vi "Ustaw wspolne.vi"(7 "WaveformGraph in":refnum<vi>, 8 "error in (no error)":errorcluster, 10 "Bounds":T2, 11 "Array":refnum<vi>[](array[refnum])) -> (0 "error out":errorcluster, 2 "Pos Array":T1[](array[typedef]))   [LabVIEW 2014]
doc: "Ustawia wspólne elementy okien Rejestracja szybka i rejestracja wolna."
uses:
  <vilib>/Utility/miscctls.llb/LVBoundsTypeDef.ctl
  <vilib>/Utility/miscctls.llb/LVPositionTypeDef.ctl
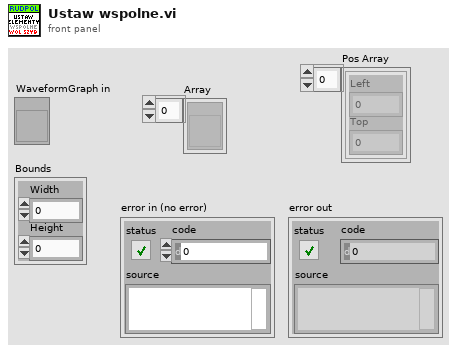
[diagram p1: front panel]
types:
  T1 = typedef "LVPositionTypeDef.ctl" = cluster{"Left":i32, "Top":i32}
  T2 = typedef "LVBoundsTypeDef.ctl" = cluster{"Width":u32, "Height":u32}
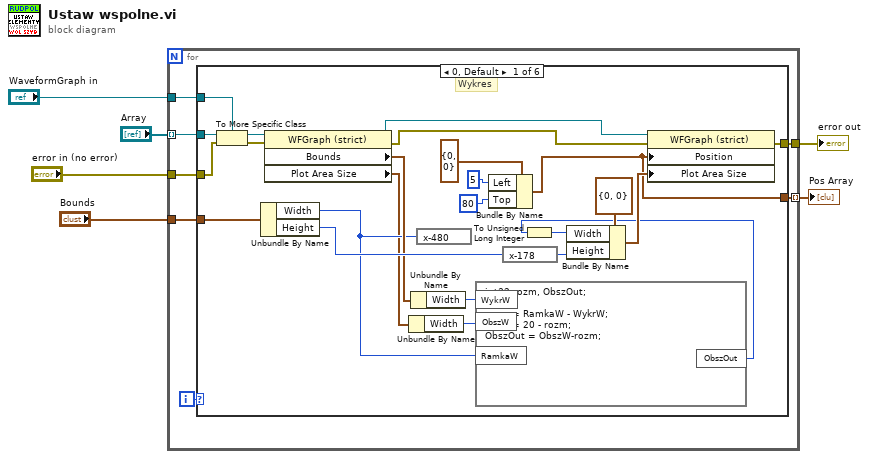
[diagram p0: block diagram]
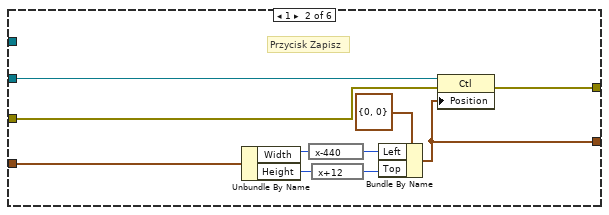
[diagram p2: hidden frame]
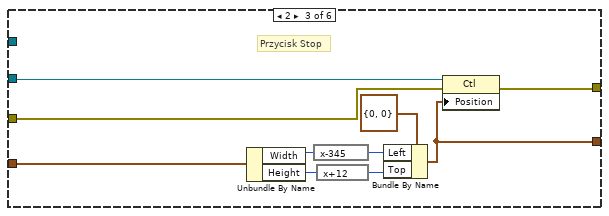
[diagram p3: hidden frame]
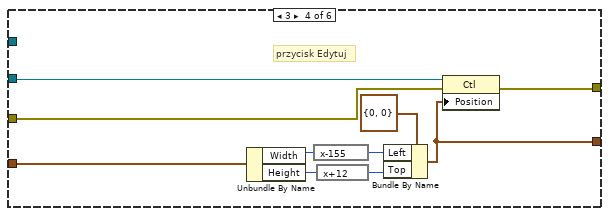
[diagram p4: hidden frame]
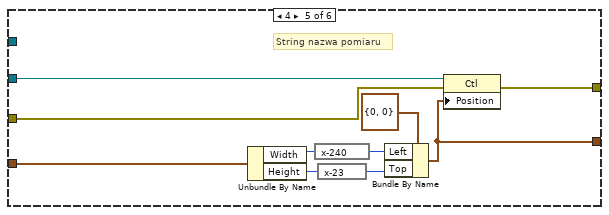
[diagram p5: hidden frame]
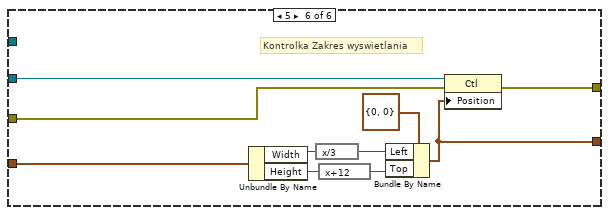
[diagram p6: hidden frame]
diagram:
  n1 = for {
    tunnel: "Array" -> [w12] mode=indexing
    tunnel: "Bounds" -> [w11]
    tunnel: "WaveformGraph in" -> [w10]
    tunnel: [w9] -> w3 mode=indexing
    tunnel: "error in (no error)" -> [w8]
    tunnel: [w7] -> w1
    i -> [w13]
    n2 = case shown="0, Default" w13 {
      tunnel: w12 -> [w34 w47 w52 w62 w72 w82]
      tunnel: w11 -> [w32 w45 w51 w61 w71 w81]
      tunnel: w10 -> [w33 _ _ _ _ _]
      tunnel: [w27 w40 w50 w60 w70 w80] -> w9
      tunnel: w8 -> [w25 w38 w48 w58 w68 w79]
      tunnel: [w26 w39 w49 w59 w69 w78] -> w7
      frame 0, Default {
        # "Wykres"
        n3 = To More Specific Class(target class=w33, reference=w34, error in=w25) -> (specific class reference=w23:refnum<vi>, error out=w24:errorcluster)
        n4 = Unbundle By Name(w32) -> ("Width"=w16:u32, "Height"=w30:u32)
        n5 = property class="WFGraph (strict)"(reference=w23, error in=w24) -> (reference out=w21:refnum<vi>, error out=w22:errorcluster, "Bounds"=w20:T2, "Plot Area Size"=w14:T2)
        n6 = Unbundle By Name(w14) -> ("Width"=w15:u32)
        n7 = Unbundle By Name(w20) -> ("Width"=w19:u32)
        n8 = expression code="x-480"(w16) -> ()  [unwired: 1 out]
        n9 = formula code="int32 rozm, ObszOut;\n\nrozm = RamkaW - WykrW;\nrozm = 20 - rozm;\nObszOut = ObszW-rozm;"("RamkaW"=w16, "WykrW"=w19, "ObszW"=w15) -> ("ObszOut"=w18:i32)
        n10 = Bundle By Name(cluster=T1 {"Left"=0, "Top"=0} ("Position"), "Left"=5 ("y"), "Top"=80 ("y")) -> (w27:T1)
        n11 = expression code="x-178"(w30) -> (w29:u32)
        n12 = To Unsigned Long Integer(number=w18) -> (unsigned 32bit integer=w17:u32)
        n13 = Bundle By Name(cluster=T2 {"Width"=0, "Height"=0} ("Plot Area:Size"), "Width"=w17, "Height"=w29) -> (w28:T2)
        n14 = property class="WFGraph (strict)"(reference=w21, error in=w22, "Position"=w27, "Plot Area Size"=w28) -> (error out=w26:errorcluster)  [unwired: 1 out]
      }
      frame 1 {
        # "Przycisk Zapisz"
        n15 = Unbundle By Name(w45) -> ("Width"=w44:u32, "Height"=w41:u32)
        n16 = expression code="x-440"(w44) -> (w43:u32)
        n17 = expression code="x+12"(w41) -> (w42:u32)
        n18 = Bundle By Name(cluster=T1 {"Left"=0, "Top"=0} ("Position"), "Left"=w43, "Top"=w42) -> (w40:T1)
        n19 = property class="Ctl"(reference=w47, error in=w38, "Position"=w40) -> (error out=w39:errorcluster)  [unwired: 1 out]
      }
      frame 2 {
        # "Przycisk Stop"
        n20 = Unbundle By Name(w51) -> ("Width"=w56:u32, "Height"=w53:u32)
        n21 = expression code="x-345"(w56) -> (w55:u32)
        n22 = expression code="x+12"(w53) -> (w54:u32)
        n23 = Bundle By Name(cluster=T1 {"Left"=0, "Top"=0} ("Position"), "Left"=w55, "Top"=w54) -> (w50:T1)
        n24 = property class="Ctl"(reference=w52, error in=w48, "Position"=w50) -> (error out=w49:errorcluster)  [unwired: 1 out]
      }
      frame 3 {
        # "przycisk Edytuj"
        n25 = Unbundle By Name(w61) -> ("Width"=w66:u32, "Height"=w63:u32)
        n26 = expression code="x-155"(w66) -> (w65:u32)
        n27 = expression code="x+12"(w63) -> (w64:u32)
        n28 = Bundle By Name(cluster=T1 {"Left"=0, "Top"=0} ("Position"), "Left"=w65, "Top"=w64) -> (w60:T1)
        n29 = property class="Ctl"(reference=w62, error in=w58, "Position"=w60) -> (error out=w59:errorcluster)  [unwired: 1 out]
      }
      frame 4 {
        # "String nazwa pomiaru"
        n30 = Unbundle By Name(w71) -> ("Width"=w76:u32, "Height"=w73:u32)
        n31 = expression code="x-240"(w76) -> (w75:u32)
        n32 = expression code="x-23"(w73) -> (w74:u32)
        n33 = Bundle By Name(cluster=T1 {"Left"=0, "Top"=0} ("Position"), "Left"=w75, "Top"=w74) -> (w70:T1)
        n34 = property class="Ctl"(reference=w72, error in=w68, "Position"=w70) -> (error out=w69:errorcluster)  [unwired: 1 out]
      }
      frame 5 {
        # "Kontrolka Zakres wyswietlania"
        n35 = Unbundle By Name(w81) -> ("Width"=w86:u32, "Height"=w83:u32)
        n36 = expression code="x/3"(w86) -> (w85:u32)
        n37 = expression code="x+12"(w83) -> (w84:u32)
        n38 = Bundle By Name(cluster=T1 {"Left"=0, "Top"=0} ("Position"), "Left"=w85, "Top"=w84) -> (w80:T1)
        n39 = property class="Ctl"(reference=w82, error in=w79, "Position"=w80) -> (error out=w78:errorcluster)  [unwired: 1 out]
      }
    }
  }
  "error out" <- w1
  "Pos Array" <- w3
